vi "Write Write.vi"(8 "error in":errorcluster, 10 "Write?":bool, 11 "File in":refnum<class "File.lvclass">) -> (0 "error out":errorcluster, 3 "File out":refnum<class "File.lvclass">)   [LabVIEW 2013, in "File.lvclass"]
uses:
  File.lvclass
  File.lvclass/File.ctl
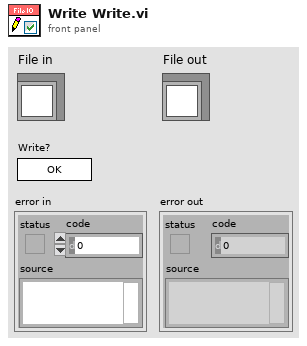
[diagram p1: front panel]
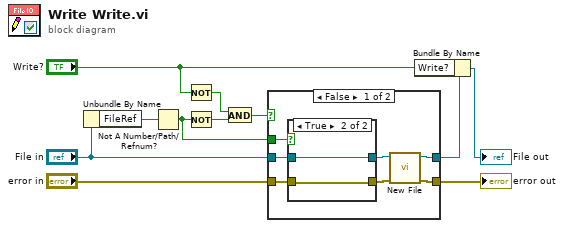
[diagram p0: block diagram]
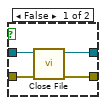
[diagram p2: hidden frame]
diagram:
  n1 = Unbundle By Name("File in") -> ("FileRef"=w7:refnum<file>)
  n2 = Not A Number/Path/Refnum?(number/path/refnum=w7) -> (NaN/Path/Refnum?=w6:bool)
  n3 = Not(x="Write?") -> (.not. x?=w9:bool)
  n4 = Not(x=w6) -> (.not. x?=w10:bool)
  n5 = And(x=w9, y=w10) -> (x .and. y?=w8:bool)
  n6 = case shown="False" w8 {
    tunnel: w6 -> [w18 _]
    tunnel: "File in" -> [w17 w26]
    tunnel: [w15 w26] -> w4
    tunnel: "error in" -> [w14 w25]
    tunnel: [w12 w25] -> w1
    frame False {
      n7 = case shown="True" w18 {
        tunnel: w17 -> [w22 w24]
        tunnel: [w21 w24] -> w16
        tunnel: w14 -> [w20 w23]
        tunnel: [w19 w23] -> w13
        frame False {
          n8 = call-dynamic "Close File.vi"("error in"=w20, "File in"=w22) -> ("error out"=w19:errorcluster, "File out"=w21:refnum<class "File.lvclass">)  [unwired: 8 in]
        }
        frame True {
        }
      }
      n9 = call-dynamic "New File.vi"("error in"=w13, "File in"=w16) -> ("error out"=w12:errorcluster, "File out"=w15:refnum<class "File.lvclass">)  [unwired: 8 in]
    }
    frame True {
    }
  }
  "error out" <- w1
  n10 = Bundle By Name(cluster=w4, "Write?"="Write?") -> (→"File out":refnum<class "File.lvclass">)
